vi "Mensaje to Hardware.vi"(8 "error in (no error)":errorcluster, 10 "Mensaje":string, 11 "UI in":refnum<class "UI.lvclass">) -> (0 "error out":errorcluster, 3 "UI out":refnum<class "UI.lvclass">)   [LabVIEW 2020, in "UI.lvlib" / "UI.lvclass"]
uses:
  UI.lvclass
  UI.lvclass/UI.ctl
  Hardware Messages/Obtain Mensaje from UI Msg/Obtain Mensaje from UI Msg.lvclass/Obtain Mensaje from UI Msg.ctl
  <vilib>/ActorFramework/Message Enqueuer/Message Enqueuer.lvclass/Message Enqueuer.ctl
  <vilib>/ActorFramework/Message Enqueuer/Enqueue.vi
  Hardware Messages/Obtain Mensaje from UI Msg/Obtain Mensaje from UI Msg.lvclass
  C:/Program Files (x86)/National Instruments/LabVIEW 2020/vi.lib/ActorFramework/Message/Message.lvclass
  <vilib>/ActorFramework/Message Priority Queue/Priority Enqueue.vi
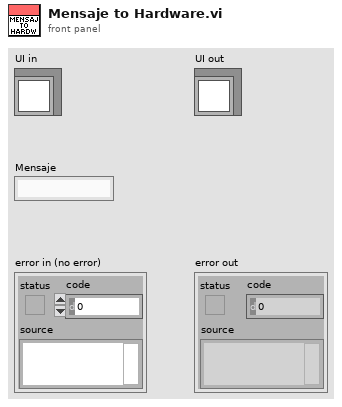
[diagram p1: front panel]
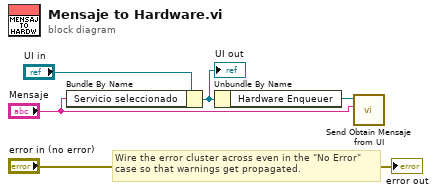
[diagram p0: block diagram]
diagram:
  # "Wire the error cluster across even in the \"No Error\"\ncase so that warnings get propagated."
  n1 = Bundle By Name(cluster="UI in", "Servicio seleccionado"="Mensaje") -> (w2:refnum<class "UI.lvclass">)
  "UI out" <- w2
  n2 = Unbundle By Name(w2) -> ("Hardware Enqueuer"=w1:refnum<class "Message Enqueuer.lvclass">)
  n3 = call "Send Obtain Mensaje from UI.vi"("Servicio seleccionado"="Mensaje", "Message Enqueuer"=w1) -> ()  [unwired: 8 in, 2 out]
  "error out" <- "error in (no error)"
